vi "feb03-sine.vi"() -> ()   [LabVIEW 2014]
uses:
  <vilib>/imath/engines/lvmath2/RunTimeEngine/Managers/WorkSpace/UID Generator.vi
  <vilib>/imath/engines/lvmath2/RunTimeEngine/RunTimeType/NIMS_RunTimeType_From StrictType (excl LVString).vi
  <instcachedir>/0/NIMS_RunTimeType_From StrictType (excl LVString)_15A5391EEA9C4AACB9955AC755B83D29.lvgen/NIMS_RunTimeType_From StrictType (excl LVString)_15A5391EEA9C4AACB9955AC755B83D29_000.vi
  <vilib>/imath/engines/lvmath2/RunTimeEngine/LocalVariableDefStatement/MC_LocalVariableDefStatement_Display.vi
  <vilib>/imath/engines/lvmath2/RunTimeEngine/RangeToken/NIMS_Range.vi
  <instcachedir>/0/NIMS_Range_9BCE657718DF4976A877346C61F22738.lvgen/NIMS_Range_9BCE657718DF4976A877346C61F22738_000.vi
  <vilib>/imathl/engines/lvmath/Functions/Error Handling/Create Error.vi
  <vilib>/imath/engines/lvmath2/RunTimeEngine/Managers/SymbolTable/Clear UID.vi
  <vilib>/imath/engines/lvmath2/RunTimeEngine/NodeEndStatement/NIMS_NodeEndStatement_Output.vi
  <instcachedir>/0/NIMS_NodeEndStatement_Output_53EC0D466D134D7ABD903AC30B43404B.lvgen/NIMS_NodeEndStatement_Output_53EC0D466D134D7ABD903AC30B43404B_001.vi
  <instcachedir>/0/NIMS_NodeEndStatement_Output_53EC0D466D134D7ABD903AC30B43404B.lvgen/NIMS_NodeEndStatement_Output_53EC0D466D134D7ABD903AC30B43404B_005.vi
  <vilib>/imath/engines/lvmath2/RunTimeEngine/ErrorHandling/NIMS_Finalize Error.vi
  <vilib>/imath/engines/lvmath2/RunTimeEngine/Managers/SymbolTable/NIMS_WorkSpace.lvlib
panel:
  out "Point per cycle":dbl
  out "x":dbl[](array[numeric])
  out "time":dbl[](array[numeric])
  out "XY Graph":cluster{"t":dbl[], "x":dbl[]}(graph)
  in  "Amplitude":dbl
  in  "sampling frequency (Hz)":dbl
  in  "f, frequency, Hz":dbl
  in  "N, num samples":i32
  # "I want to have an indicator that\ngives points per cycle of the wave.  \nPlease fix this vi."
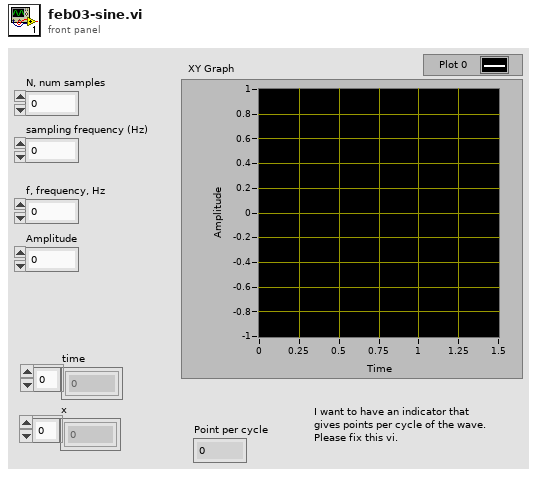
[diagram p1: front panel]
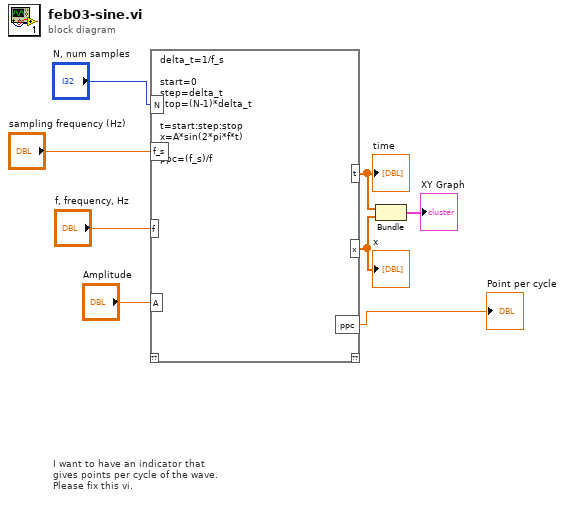
[diagram p0: block diagram]
diagram:
  # "I want to have an indicator that\ngives points per cycle of the wave.  \nPlease fix this vi."
  n1 = mathscript code="delta_t=1/f_s\n\nstart=0\nstep=delta_t\nstop=(N-1)*delta_t\n\nt=start:step:stop\nx=A*sin(2*pi*f*t)\n\nppc=(f_s)/f"("N"="N, num samples", "f_s"="sampling frequency (Hz)", "f"="f, frequency, Hz", "A"="Amplitude") -> ("t"=w4:dbl[], "x"=w3:dbl[], "ppc"=→"Point per cycle":dbl)  [unwired: 1 in, 1 out]
  "time" <- w4
  "x" <- w3
  n2 = Bundle("t"=w4, "x"=w3) -> (→"XY Graph":cluster{"t":dbl[], "x":dbl[]})  [unwired: 1 in]
